vi "Coffee_Machine_Producer_Consumer_Loop.vi"() -> ()   [LabVIEW 2014]
uses:
  States.ctl
panel:
  out "Elapsed Time (s)":dbl
  out "Now Vending":T1
  out "Vending Progress":u8(slide) scale=0.0..100.0
  in  "stop":bool
  out "Coffee Out?":bool
  out "Water Out?":bool
  out "Tea Out?":bool
  out "Milk Out?":bool
  in  "Tea":bool
  in  "Coffee":bool
  in  "Milk":bool
  out "Water  (ml)":u32(slide) scale=0.0..10000.0
  out "Tea Powder (gms)":u32(slide) scale=0.0..10000.0
  out "Coffee Powder (gms)":u32(slide) scale=0.0..10000.0
  out "Milk (ml)":u32(slide) scale=0.0..10000.0
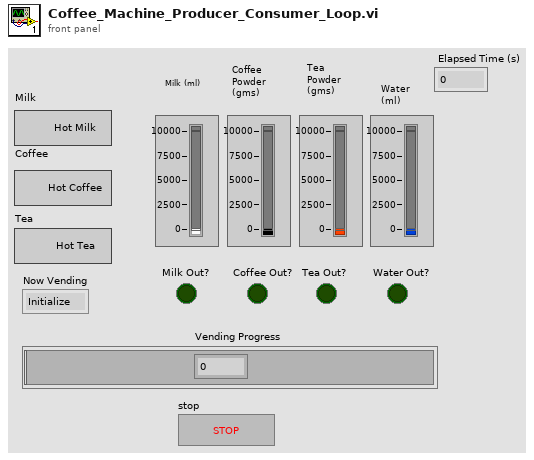
[diagram p1: front panel]
types:
  T1 = typedef "States.ctl" = enum16{"Initialize", "Default", "Milk", "Coffee", "Tea", "Progress", "Shutdown"}
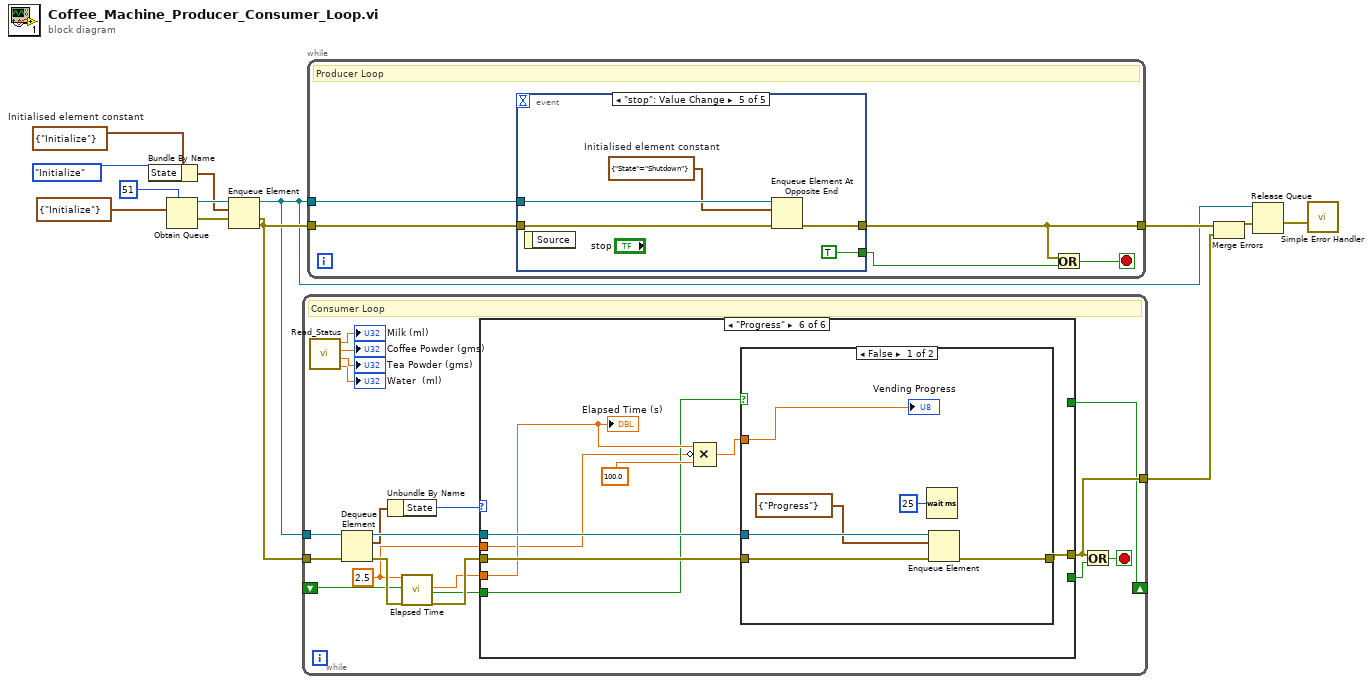
[diagram p0: block diagram]
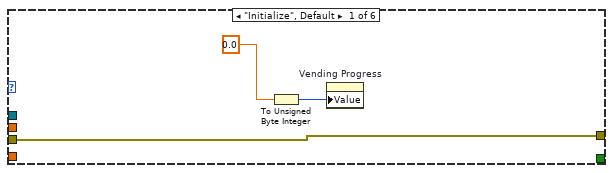
[diagram p2: hidden frame]
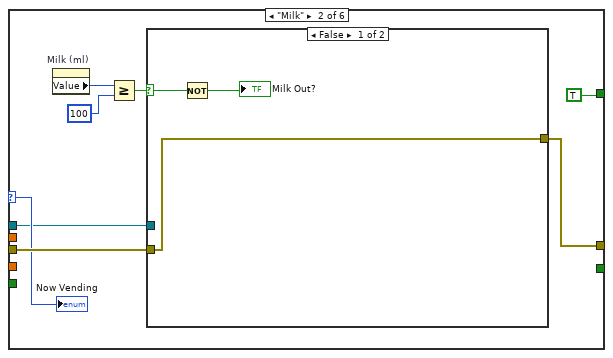
[diagram p3: hidden frame]
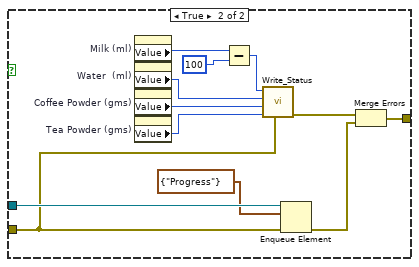
[diagram p4: hidden frame]
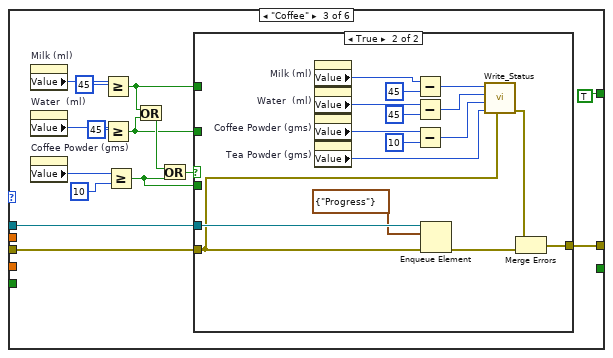
[diagram p5: hidden frame]
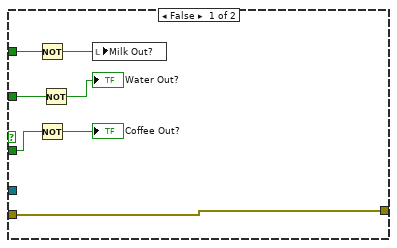
[diagram p6: hidden frame]
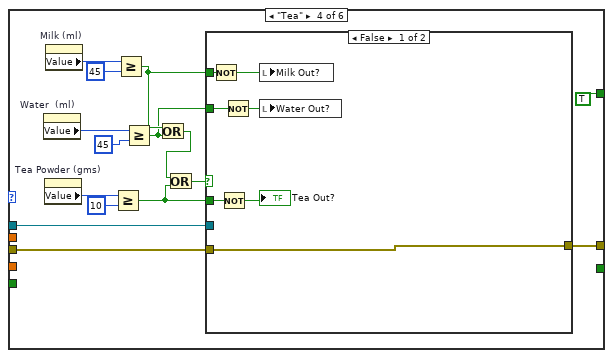
[diagram p7: hidden frame]
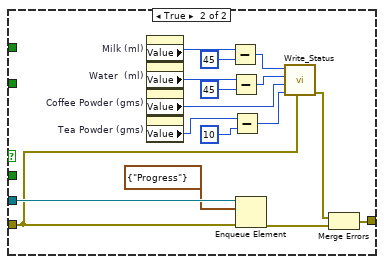
[diagram p8: hidden frame]
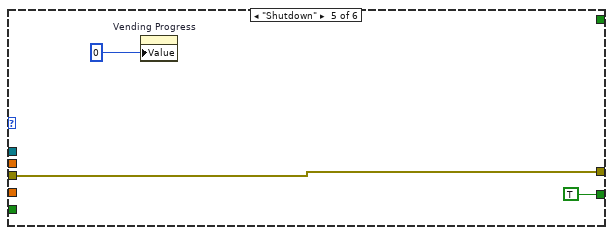
[diagram p9: hidden frame]
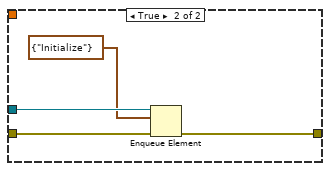
[diagram p10: hidden frame]
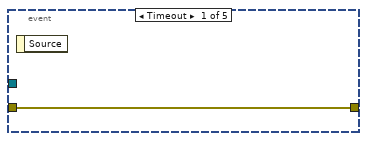
[diagram p11: hidden frame]
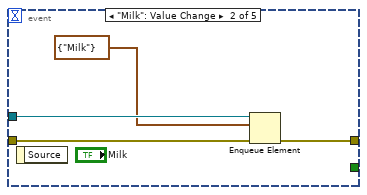
[diagram p12: hidden frame]
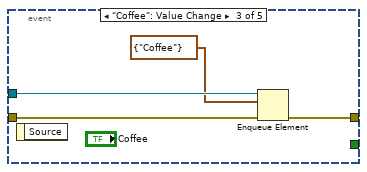
[diagram p13: hidden frame]
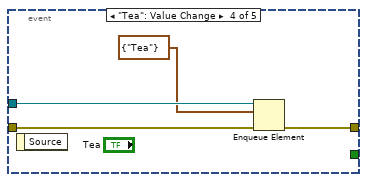
[diagram p14: hidden frame]
diagram:
  w13 = cluster{"State":T1} {"State"=enum."Initialize"}  # Initialised element constant
  n1 = Bundle By Name(cluster=w13, "State"=States."Initialize") -> (w10:cluster{"State":T1})
  n2 = Obtain Queue(max queue size (-1, unlimited)=51, element data type=cluster{"State":T1} {"State"=enum."Initialize"} ("Initialised element constant")) -> (queue out=w12:refnum<queue>, error out=w11:errorcluster)  [unwired: 3 in, 1 out]
  n3 = Enqueue Element(queue=w12, element=w10, error in (no error)=w11) -> (queue out=w3:refnum<queue>, error out=w4:errorcluster)  [unwired: 1 in, 1 out]
  n4 = while "Consumer Loop" {
    tunnel: w3 -> [w31]
    tunnel: w4 -> [w30]
    tunnel: [w25] -> w2
    shift-right: [w20] -> _
    shift-left: _ -> [w17]
    stop <- w27 stop-if-true
    w14 = 2.5 ("Time Target (s)")
    # "Consumer Loop"
    n5 = call "Read_Status.vi"() -> ("Water\n   (Lt)"=→"Water  (ml)":dbl, "Tea Powder\n       (Kg)"=→"Tea Powder (gms)":dbl, "Coffee Powder\n         (Kg)"=→"Coffee Powder (gms)":dbl, "Milk\n (Lt)"=→"Milk (ml)":dbl)  [unwired: 8 in]
    n6 = Dequeue Element(queue=w31, error in (no error)=w30) -> (queue out=w32:refnum<queue>, element=w29:cluster{"State":T1}, error out=w19:errorcluster)  [unwired: 1 in, 1 out]
    n7 = Unbundle By Name(w29) -> ("State"=w28:T1)
    n8 = call "Elapsed Time"("Time Target (s)"=w14, "Reset"=w17, "error in (no error)"=w19) -> ("Elapsed Time (s)"=w16:dbl, "Time has Elapsed"=w15:bool, "error out"=w18:errorcluster)  [unwired: 9 in, 5 out]
    n9 = case shown="\"Progress\"" w28 {
      selector: w28 -> [_ w38 _ _ _ _]
      tunnel: w18 -> [w35 w40 w65 w111 w137 w141]
      tunnel: [w35 w39 w64 w110 w137 w144] -> w25
      tunnel: [_ _ _ _ TRUE _] -> w26
      tunnel: w32 -> [_ w37 w63 w101 _ w145]
      tunnel: [_ TRUE TRUE TRUE _ _] -> w20
      tunnel: w16 -> [_ _ _ _ _ w140]
      tunnel: w15 -> [_ _ _ _ _ w139]
      tunnel: w14 -> [_ _ _ _ _ w138]
      frame "Initialize", Default {
        n10 = To Unsigned Byte Integer(number=0.0 ("Percentage")) -> (unsigned 8bit integer=w33:u8)
        n11 = property on="Vending Progress" class="Slide (strict)"("Value"=w33) -> ()  [unwired: 2 in, 2 out]
      }
      frame "Milk" {
        n12 = property on="Milk (ml)" class="Slide (strict)"() -> ("Value"=w42:u32)  [unwired: 2 in, 2 out]
        n13 = Greater Or Equal?(x=w42, y=u32 100) -> (x >= y?=w43:bool)
        n14 = case shown="False" w43 {
          selector: w43 -> [w45 _]
          tunnel: w40 -> [w46 w50]
          tunnel: [w46 w49] -> w39
          tunnel: w37 -> [_ w52]
          frame False {
            n15 = Not(x=w45) -> (.not. x?=→"Milk Out?":bool)
          }
          frame True {
            n16 = property on="Milk (ml)" class="Slide (strict)"() -> ("Value"=w54:u32)  [unwired: 2 in, 2 out]
            n17 = property on="Water  (ml)" class="Slide (strict)"() -> ("Value"=w56:u32)  [unwired: 2 in, 2 out]
            n18 = property on="Coffee Powder (gms)" class="Slide (strict)"() -> ("Value"=w58:u32)  [unwired: 2 in, 2 out]
            n19 = property on="Tea Powder (gms)" class="Slide (strict)"() -> ("Value"=w57:u32)  [unwired: 2 in, 2 out]
            n20 = Subtract(x=w54, y=u32 100) -> (x-y=w55:u32)
            n21 = call "Write_Status.vi"("Error In"=w50, "Tea Powder\n       (Kg)"=w57, "Coffee Powder\n         (Kg)"=w58, "Water\n   (Lt)"=w56, "Milk\n (Lt)"=w55) -> ("Error Out"=w48:errorcluster)  [unwired: 6 in]
            n22 = Enqueue Element(queue=w52, element=cluster{"State":T1} {"State"=enum."Progress"}, error in (no error)=w50) -> (error out=w47:errorcluster)  [unwired: 1 in, 2 out]
            n23 = Merge Errors(w48, w47) -> (w49:errorcluster)
          }
        }
        "Now Vending" <- w38
      }
      frame "Coffee" {
        n24 = property on="Milk (ml)" class="Slide (strict)"() -> ("Value"=w73:u32)  [unwired: 2 in, 2 out]
        n25 = property on="Water  (ml)" class="Slide (strict)"() -> ("Value"=w72:u32)  [unwired: 2 in, 2 out]
        n26 = property on="Coffee Powder (gms)" class="Slide (strict)"() -> ("Value"=w71:u32)  [unwired: 2 in, 2 out]
        n27 = Greater Or Equal?(x=w73, y=u32 45) -> (x >= y?=w61:bool)
        n28 = Greater Or Equal?(x=w72, y=u32 45) -> (x >= y?=w60:bool)
        n29 = Greater Or Equal?(x=w71, y=u32 10) -> (x >= y?=w59:bool)
        n30 = Or(x=w61, y=w60) -> (x .or. y?=w66:bool)
        n31 = Or(x=w66, y=w59) -> (x .or. y?=w67:bool)
        n32 = case shown="True" w67 {
          tunnel: w65 -> [w80 w85]
          tunnel: [w80 w84] -> w64
          tunnel: w63 -> [_ w86]
          tunnel: w61 -> [w79 _]
          tunnel: w60 -> [w78 _]
          tunnel: w59 -> [w77 _]
          frame False {
            n33 = Not(x=w79) -> (.not. x?=w76:bool)
            n34 = Not(x=w77) -> (.not. x?=→"Coffee Out?":bool)
            n35 = Not(x=w78) -> (.not. x?=→"Water Out?":bool)
            n36 = local write "Milk Out?"(w76) -> ()
          }
          frame True {
            n37 = property on="Milk (ml)" class="Slide (strict)"() -> ("Value"=w96:u32)  [unwired: 2 in, 2 out]
            n38 = property on="Water  (ml)" class="Slide (strict)"() -> ("Value"=w95:u32)  [unwired: 2 in, 2 out]
            n39 = property on="Coffee Powder (gms)" class="Slide (strict)"() -> ("Value"=w94:u32)  [unwired: 2 in, 2 out]
            n40 = property on="Tea Powder (gms)" class="Slide (strict)"() -> ("Value"=w93:u32)  [unwired: 2 in, 2 out]
            n41 = Subtract(x=w96, y=u32 45) -> (x-y=w89:u32)
            n42 = Subtract(x=w95, y=u32 45) -> (x-y=w88:u32)
            n43 = Subtract(x=w94, y=u32 10) -> (x-y=w87:u32)
            n44 = Enqueue Element(queue=w86, element=cluster{"State":T1} {"State"=enum."Progress"}, error in (no error)=w85) -> (error out=w82:errorcluster)  [unwired: 1 in, 2 out]
            n45 = call "Write_Status.vi"("Error In"=w85, "Tea Powder\n       (Kg)"=w93, "Coffee Powder\n         (Kg)"=w87, "Water\n   (Lt)"=w88, "Milk\n (Lt)"=w89) -> ("Error Out"=w83:errorcluster)  [unwired: 6 in]
            n46 = Merge Errors(w83, w82) -> (w84:errorcluster)
          }
        }
      }
      frame "Tea" {
        n47 = property on="Water  (ml)" class="Slide (strict)"() -> ("Value"=w108:u32)  [unwired: 2 in, 2 out]
        n48 = property on="Tea Powder (gms)" class="Slide (strict)"() -> ("Value"=w107:u32)  [unwired: 2 in, 2 out]
        n49 = property on="Milk (ml)" class="Slide (strict)"() -> ("Value"=w109:u32)  [unwired: 2 in, 2 out]
        n50 = Greater Or Equal?(x=w107, y=u32 10) -> (x >= y?=w97:bool)
        n51 = Greater Or Equal?(x=w109, y=u32 45) -> (x >= y?=w99:bool)
        n52 = Greater Or Equal?(x=w108, y=u32 45) -> (x >= y?=w98:bool)
        n53 = Or(x=w99, y=w98) -> (x .or. y?=w102:bool)
        n54 = Or(x=w102, y=w97) -> (x .or. y?=w103:bool)
        n55 = case shown="False" w103 {
          tunnel: w111 -> [w118 w123]
          tunnel: [w118 w122] -> w110
          tunnel: w101 -> [_ w124]
          tunnel: w99 -> [w117 _]
          tunnel: w98 -> [w116 _]
          tunnel: w97 -> [w115 _]
          frame False {
            n56 = Not(x=w117) -> (.not. x?=w114:bool)
            n57 = Not(x=w115) -> (.not. x?=→"Tea Out?":bool)
            n58 = Not(x=w116) -> (.not. x?=w113:bool)
            n59 = local write "Milk Out?"(w114) -> ()
            n60 = local write "Water Out?"(w113) -> ()
          }
          frame True {
            n61 = property on="Milk (ml)" class="Slide (strict)"() -> ("Value"=w133:u32)  [unwired: 2 in, 2 out]
            n62 = property on="Water  (ml)" class="Slide (strict)"() -> ("Value"=w131:u32)  [unwired: 2 in, 2 out]
            n63 = property on="Coffee Powder (gms)" class="Slide (strict)"() -> ("Value"=w130:u32)  [unwired: 2 in, 2 out]
            n64 = property on="Tea Powder (gms)" class="Slide (strict)"() -> ("Value"=w129:u32)  [unwired: 2 in, 2 out]
            n65 = Subtract(x=w133, y=u32 45) -> (x-y=w134:u32)
            n66 = Subtract(x=w131, y=u32 45) -> (x-y=w132:u32)
            n67 = Subtract(x=w129, y=u32 10) -> (x-y=w128:u32)
            n68 = Enqueue Element(queue=w124, element=cluster{"State":T1} {"State"=enum."Progress"}, error in (no error)=w123) -> (error out=w121:errorcluster)  [unwired: 1 in, 2 out]
            n69 = call "Write_Status.vi"("Error In"=w123, "Tea Powder\n       (Kg)"=w128, "Coffee Powder\n         (Kg)"=w130, "Water\n   (Lt)"=w132, "Milk\n (Lt)"=w134) -> ("Error Out"=w120:errorcluster)  [unwired: 6 in]
            n70 = Merge Errors(w120, w121) -> (w122:errorcluster)
          }
        }
      }
      frame "Shutdown" {
        n71 = property on="Vending Progress" class="Slide (strict)"("Value"=u8 0 ("Vending Progress")) -> ()  [unwired: 2 in, 2 out]
      }
      frame "Progress" {
        n72 = Compound Arithmetic op=MULTIPLY(w140, invert w138, 100.0 ("Time Target (s)")) -> (w142:dbl)
        n73 = case shown="False" w139 {
          tunnel: w145 -> [w151 w153]
          tunnel: w141 -> [w147 w155]
          tunnel: [w150 w154] -> w144
          tunnel: w142 -> [w146 _]
          frame False {
            n74 = Wait (ms)(milliseconds to wait=u32 25) -> ()  [unwired: 1 out]
            n75 = Enqueue Element(queue=w151, element=cluster{"State":T1} {"State"=enum."Progress"}, error in (no error)=w147) -> (error out=w150:errorcluster)  [unwired: 1 in, 2 out]
            "Vending Progress" <- w146
          }
          frame True {
            n76 = Enqueue Element(queue=w153, element=cluster{"State":T1} {"State"=enum."Initialize"}, error in (no error)=w155) -> (error out=w154:errorcluster)  [unwired: 1 in, 2 out]
          }
        }
        "Elapsed Time (s)" <- w140
      }
    }
    n77 = Or(x=w25, y=w26) -> (x .or. y?=w27:bool)
  }
  n78 = while "Producer Loop" {
    tunnel: w3 -> [w160]
    tunnel: w4 -> [w159]
    tunnel: [w157] -> w5
    stop <- w158 stop-if-true
    # "Producer Loop"
    n79 = event shown="[4] \"stop\": Value Change" {
      selector: _ -> [_ _ _ _ _]
      dyn-events: _ -> [_ _ _ _ _]
      timeout: _ -> [_ _ _ _ _]
      tunnel: w160 -> [_ w165 w167 w171 w175]
      tunnel: w159 -> [w161 w164 w168 w172 w176]
      tunnel: [w161 w163 w169 w173 w177] -> w157
      tunnel: [_ _ _ _ TRUE] -> w156
      event Timeout {
        n80 = event-data() -> ()  [unwired: 1 in, 1 out]
      }
      event "Milk": Value Change {
        n81 = event-data() -> ()  [unwired: 1 in, 1 out]
        n82 = Enqueue Element(queue=w165, element=cluster{"State":T1} {"State"=enum."Milk"} ("Initialised element constant"), error in (no error)=w164) -> (error out=w163:errorcluster)  [unwired: 1 in, 2 out]
      }
      event "Coffee": Value Change {
        n83 = event-data() -> ()  [unwired: 1 in, 1 out]
        n84 = Enqueue Element(queue=w167, element=cluster{"State":T1} {"State"=enum."Coffee"} ("Initialised element constant"), error in (no error)=w168) -> (error out=w169:errorcluster)  [unwired: 1 in, 2 out]
      }
      event "Tea": Value Change {
        n85 = event-data() -> ()  [unwired: 1 in, 1 out]
        n86 = Enqueue Element(queue=w171, element=cluster{"State":T1} {"State"=enum."Tea"} ("Initialised element constant"), error in (no error)=w172) -> (error out=w173:errorcluster)  [unwired: 1 in, 2 out]
      }
      event "stop": Value Change {
        w174 = cluster{"State":T1} {"State"=enum."Shutdown"}  # Initialised element constant
        n87 = event-data() -> ()  [unwired: 1 in, 1 out]
        n88 = Enqueue Element At Opposite End(queue=w175, element=w174, error in (no error)=w176) -> (error out=w177:errorcluster)  [unwired: 1 in, 2 out]
      }
    }
    n89 = Or(x=w157, y=w156) -> (x .or. y?=w158:bool)
  }
  n90 = Merge Errors(w5, w2) -> (w7:errorcluster)
  n91 = Release Queue(queue=w3, error in (no error)=w7) -> (error out=w6:errorcluster)  [unwired: 1 in, 2 out]
  n92 = call <vilib>:"Simple Error Handler.vi"("error in (no error)"=w6) -> ()  [unwired: 4 in, 5 out]
